vi "Serial Read with Timeout.vi"(6 "Error In (no error)":errorcluster, 8 "Timeout Limit":dbl=5.0 format="%.2f", 9 "Resource Name":refnum<visa-resource-name>="ASRL1::INSTR") -> (0 "Error Out":errorcluster, 1 "Serial Settings:Number of Bytes at Serial Port":u32, 2 "Serial Read":string, 3 "Dup VISA Resource Name":refnum<visa-resource-name>)   [LabVIEW 2011]
doc: "The Serial Read with Timeout VI will read bytes until either the requested number of bytes is received, or until a timeout occurs."
panel:
  # "Select or enter the serial resource."
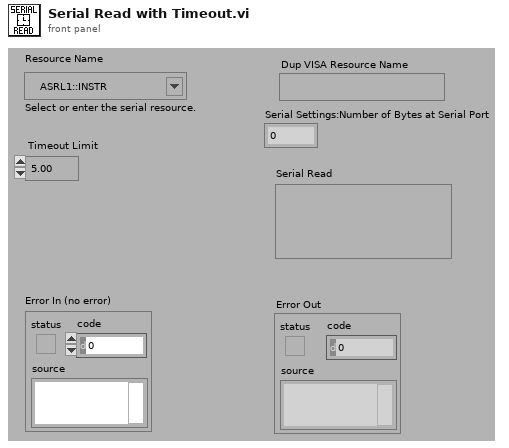
[diagram p1: front panel]
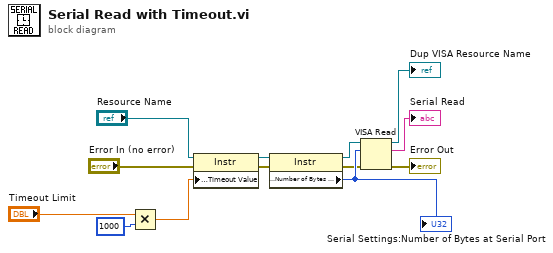
[diagram p0: block diagram]
diagram:
  n1 = Multiply(x="Timeout Limit", y=1000) -> (x*y=w11:dbl)
  n2 = property class="Instr"(reference="Resource Name", error in="Error In (no error)", "General Settings:Timeout Value"=w11) -> (reference out=w5:refnum<visa-resource-name>, error out=w4:errorcluster)
  n3 = property class="Instr"(reference=w5, error in=w4) -> (reference out=w2:refnum<visa-resource-name>, error out=w1:errorcluster, "Serial Settings:Number of Bytes at Serial Port"=w3:u32)
  "Serial Settings:Number of Bytes at Serial Port" <- w3
  n4 = VISA Read(VISA resource name=w2, byte count=w3, error in (no error)=w1) -> (VISA resource name out=→"Dup VISA Resource Name":refnum<visa-resource-name>, read buffer=→"Serial Read":string, error out=→"Error Out":errorcluster)  [unwired: 1 out]
